vi "Read value (String).vi"(8 "error in (no error)":errorcluster, 9 "default value":string, 11 "JSON String in":refnum<class "JSON Value.lvclass">) -> (0 "error out":errorcluster, 1 "defaulted?":bool, 2 "value":string)   [LabVIEW 2016, in "JSON Value.lvclass"]
doc: "Returns the value of a JSON String"
uses:
  JSON Value.lvclass
  JSON Value.lvclass/JSON Value.ctl
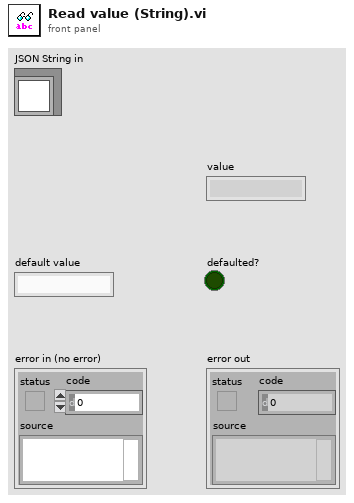
[diagram p1: front panel]
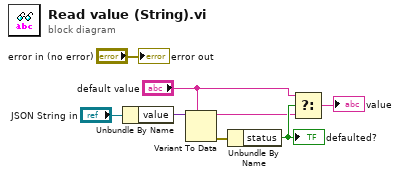
[diagram p0: block diagram]
diagram:
  n1 = Unbundle By Name("JSON String in") -> ("value"=w3:variant)
  n2 = Variant To Data(type="default value", Variant=w3) -> (data=w2:string, error out=w1:errorcluster)  [unwired: 1 in]
  n3 = Unbundle By Name(w1) -> ("status"=w4:bool)
  "defaulted?" <- w4
  n4 = Select(t="default value", s=w4, f=w2) -> (s? t:f=→"value":string)
  "error out" <- "error in (no error)"
